vi "CRYInsert Sequence Data.vi"(8 "sOption":string, 9 "New Step No.":i32[](array[numeric]), 10 "Old Step No.":i32[](array[numeric]), 11 "sFlattenedCurveData":string) -> (2 "New Names Out":string[](array[string]), 3 "Old Names Out":string[](array[string]))   [LabVIEW 2013]
panel:
  # "Insert Sequence Data"
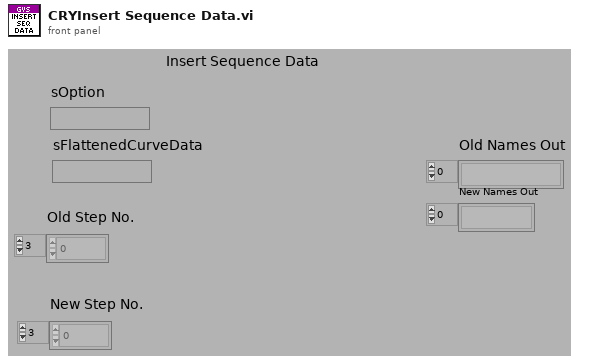
[diagram p1: front panel]
types:
  T1 = typedef "CRYCurve Library Cluster.ctl" = cluster{"Curves":T2, "Results":T4, "Values":T2, "Waveforms":T6, "Curve Items":cluster{"Left Cell String":string, "Child Text":string[], "Child Tag":string, "Item Indent":i32, "Child Only?":bool, "Glyph Index":i32}[], "Value Items":cluster{"Left Cell String":string, "Child Text":string[], "Child Tag":string, "Item Indent":i32, "Child Only?":bool, "Glyph Index":i32}[], "Result Items":cluster{"Left Cell String":string, "Child Text":string[], "Child Tag":string, "Item Indent":i32, "Child Only?":bool, "Glyph Index":i32}[], "WFM Items":cluster{"Left Cell String":string, "Child Text":string[], "Child Tag":string, "Item Indent":i32, "Child Only?":bool, "Glyph Index":i32}[]}
  T2 = typedef "CRYData Cluster Array.ctl" = T3[]
  T3 = typedef "CRYData Cluster.ctl" = cluster{"Name":string, "Curve":cluster{"x":dbl, "y":dbl, "z":dbl}[], "X data":u16, "Y data":u16, "Z data":u16, "X axis":u16, "Y axis":u16, "Z axis":u16, "X unit":string, "Y unit":string, "Z unit":string, "X dB ref":dbl, "Y dB ref":dbl, "Z dB ref":dbl, "single val":bool, "protected":bool, "display X":bool, "display Y":bool, "display Z":bool, "Test Info":string, "Step No.":i32, "Plot Settings":cluster{"Color":u32, "Interpolation":u8, "Point Style":u8, "Line Style":u8, "Point Color":u32, "Line Width":u8, "Bar Plot Style":u8, "Fill To":i16}, "AutoProtect":bool}
  T4 = typedef "CRYResult Cluster Array.ctl" = T5[]
  T5 = typedef "CRYResult Cluster.ctl" = cluster{"Name":string, "Margin":dbl, "unit":string, "Verdict":bool, "Limit":string, "Max/Min":string, "protected":bool, "Step No.":i32, "Test Info":string, "AutoProtect":bool}
  T6 = typedef "CRYWaveform Cluster Array.ctl" = T7[]
  T7 = typedef "CRYWaveform Cluster.ctl" = cluster{"Waveform":cluster{"X0":dbl, "dX":dbl, "Y":sgl[]}, "X data":u16, "Y data":u16, "Y axis":u16, "X unit":string, "Y unit":string, "Y dB ref":dbl, "display Y":bool, "display X":bool, "Overload?":bool, "Test Info":string, "Step No.":i32, "Name":string, "protected":bool, "Sqc history":string[], "Signal Channel ID":i32, "Plot Settings":cluster{"Color":u32, "Interpolation":u8, "Point Style":u8, "Line Style":u8, "Point Color":u32, "Line Width":u8, "Bar Plot Style":u8, "Fill To":i16}, "AutoProtect":bool}
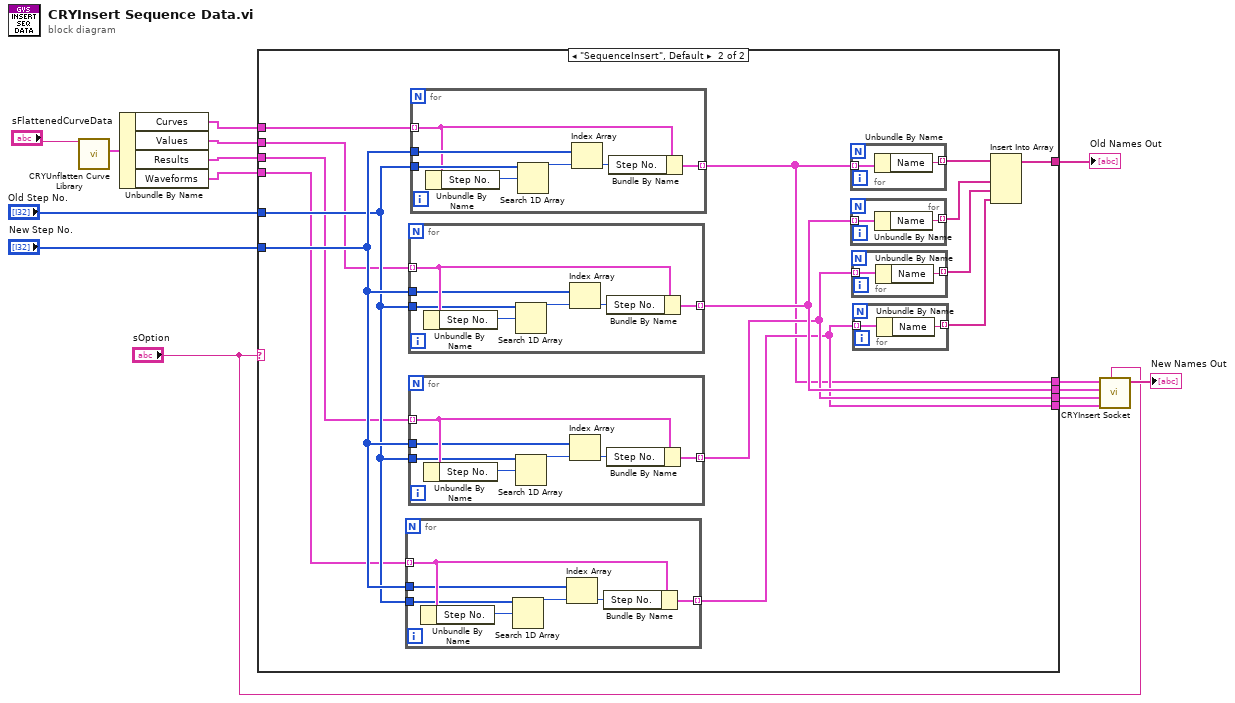
[diagram p0: block diagram]
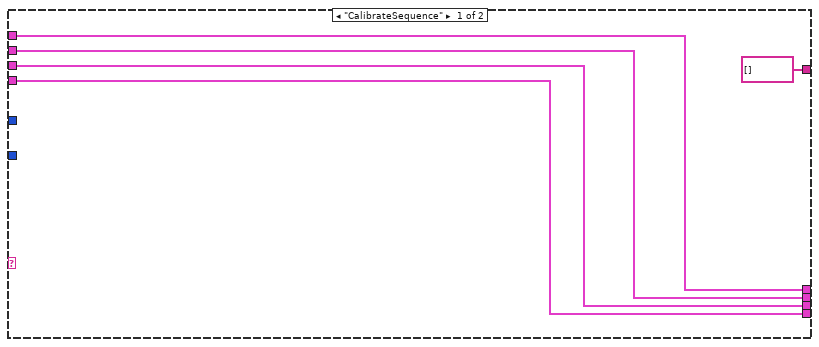
[diagram p2: hidden frame]
diagram:
  n1 = call "CRYUnflatten Curve Library.vi"("Flatten CurLib"="sFlattenedCurveData") -> ("CurLib Cluster"=w14:T1)  [unwired: 8 in, 2 out]
  n2 = Unbundle By Name(w14) -> ("Curves"=w3:T2, "Values"=w9:T2, "Results"=w7:T4, "Waveforms"=w5:T6)
  n3 = case shown="\"SequenceInsert\", Default" "sOption" {
    tunnel: [string[] [] w31] -> w13
    tunnel: "New Step No." -> [_ w30]
    tunnel: "Old Step No." -> [_ w29]
    tunnel: w9 -> [w18 w28]
    tunnel: [w18 w27] -> w8
    tunnel: w7 -> [w17 w26]
    tunnel: [w17 w25] -> w6
    tunnel: w5 -> [w16 w24]
    tunnel: [w16 w23] -> w4
    tunnel: w3 -> [w19 w22]
    tunnel: [w19 w21] -> w2
    frame "CalibrateSequence" {
    }
    frame "SequenceInsert", Default {
      n4 = for {
        tunnel: w24 -> [w42] mode=indexing
        tunnel: w29 -> [w41]
        tunnel: w30 -> [w39]
        tunnel: [w36] -> w23 mode=indexing
        n5 = Unbundle By Name(w42) -> ("Step No."=w40:i32)
        n6 = Search 1D Array(1D array=w41, element=w40) -> (index of element=w38:i32)  [unwired: 1 in]
        n7 = Index Array(array=w39, index=w38) -> (element=w37:i32)
        n8 = Bundle By Name(cluster=w42, "Step No."=w37) -> (w36:T7)
      }
      n9 = for {
        tunnel: w28 -> [w56] mode=indexing
        tunnel: w29 -> [w55]
        tunnel: w30 -> [w53]
        tunnel: [w50] -> w27 mode=indexing
        n10 = Unbundle By Name(w56) -> ("Step No."=w54:i32)
        n11 = Search 1D Array(1D array=w55, element=w54) -> (index of element=w52:i32)  [unwired: 1 in]
        n12 = Index Array(array=w53, index=w52) -> (element=w51:i32)
        n13 = Bundle By Name(cluster=w56, "Step No."=w51) -> (w50:T3)
      }
      n14 = for {
        tunnel: w26 -> [w49] mode=indexing
        tunnel: w29 -> [w48]
        tunnel: w30 -> [w46]
        tunnel: [w43] -> w25 mode=indexing
        n15 = Unbundle By Name(w49) -> ("Step No."=w47:i32)
        n16 = Search 1D Array(1D array=w48, element=w47) -> (index of element=w45:i32)  [unwired: 1 in]
        n17 = Index Array(array=w46, index=w45) -> (element=w44:i32)
        n18 = Bundle By Name(cluster=w49, "Step No."=w44) -> (w43:T5)
      }
      n19 = for {
        tunnel: w22 -> [w57] mode=indexing
        tunnel: w29 -> [w63]
        tunnel: w30 -> [w61]
        tunnel: [w58] -> w21 mode=indexing
        n20 = Unbundle By Name(w57) -> ("Step No."=w62:i32)
        n21 = Search 1D Array(1D array=w63, element=w62) -> (index of element=w60:i32)  [unwired: 1 in]
        n22 = Index Array(array=w61, index=w60) -> (element=w59:i32)
        n23 = Bundle By Name(cluster=w57, "Step No."=w59) -> (w58:T3)
      }
      n24 = for {
        tunnel: w21 -> [w71] mode=indexing
        tunnel: [w70] -> w35 mode=indexing
        n25 = Unbundle By Name(w71) -> ("Name"=w70:string)
      }
      n26 = for {
        tunnel: w27 -> [w69] mode=indexing
        tunnel: [w68] -> w34 mode=indexing
        n27 = Unbundle By Name(w69) -> ("Name"=w68:string)
      }
      n28 = for {
        tunnel: w25 -> [w67] mode=indexing
        tunnel: [w66] -> w33 mode=indexing
        n29 = Unbundle By Name(w67) -> ("Name"=w66:string)
      }
      n30 = for {
        tunnel: w23 -> [w65] mode=indexing
        tunnel: [w64] -> w32 mode=indexing
        n31 = Unbundle By Name(w65) -> ("Name"=w64:string)
      }
      n32 = Insert Into Array(array=w35, new element #1=w34, new element #2=w33, new element #3=w32) -> (w31:string[])  [unwired: 1 in]
    }
  }
  "Old Names Out" <- w13
  n33 = call "CRYInsert Socket.vi"("sOption1"="sOption", "Waves"=w4, "Results"=w6, "Values"=w8, "Curves"=w2) -> ("Inserted Names Out"=→"New Names Out":string[])  [unwired: 6 in]
